vi "example_get_wavfile_amplitudes.vi"() -> ()   [LabVIEW 2017]
uses:
  <vilib>/rvi/interface/nirviOpenFPGA/nirviOpenFPGA.xnode
  <vilib>/rvi/interface/nirviCloseFPGA/nirviCloseFPGA.xnode
  <vilib>/FPGAPlugInAG/Dynamic/niLvFpga_Close_Dynamic.vi
  <vilib>/rvi/interface/nirviMethod/nirviMethod.xnode
  <vilib>/FPGAPlugInAG/Dynamic/niLvFpga_WriteFifo_Dynamic.vi
  <vilib>/rvi/errors/niLvFpgaMergeErrorWithErrorCode.vi
  FPGA Bitfiles/lab4_FPGATarget_fpgafir_PosNEB8kOJw.lvbitx
  <vilib>/FPGAPlugInAG/myRIO-1900/niLvFpga_Open_myRIO-1900.vi
  <vilib>/rvi/interface/common/dynamic/niFpgaDynamicAddResources.vi
panel:
  out "stream chart":dbl(graph)
  out "dt":dbl
  out "Wav file Amplitude graph":dbl[](graph)
  out "t0":timestamp
  out "Waveform Graph":waveform(dbl)(graph)
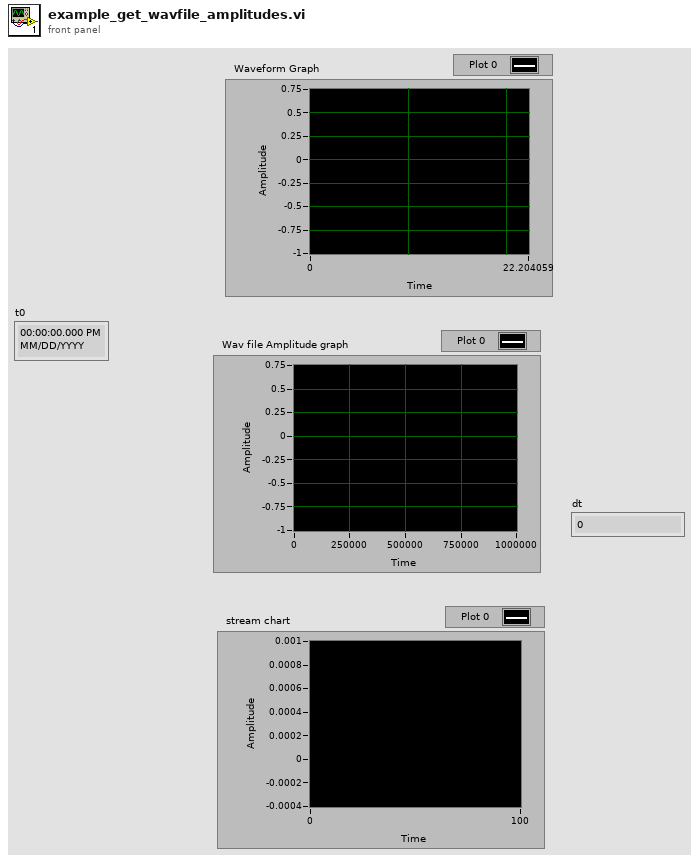
[diagram p1: front panel]
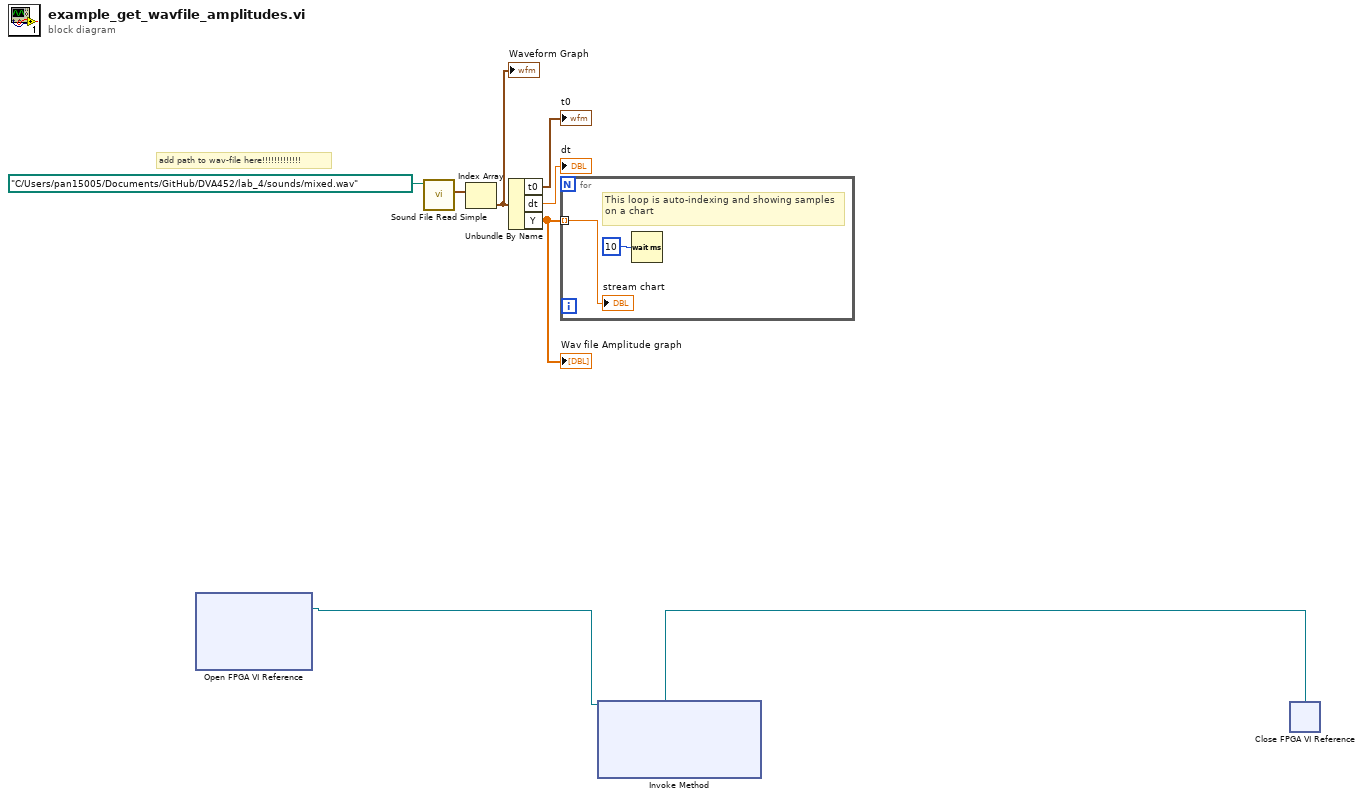
[diagram p0: block diagram]
diagram:
  # "add path to wav-file here!!!!!!!!!!!!!"
  n1 = xnode "Open FPGA VI Reference"() -> ("FPGA VI Reference Out"=w2:refnum<k20>)  [unwired: 2 in, 1 out]
  n2 = call <vilib>:"Sound File Read Simple.vi"("path"=path "C:/Users/pan15005/Documents/GitHub/DVA452/lab_4/sounds/mixed.wav") -> ("data"=w3:waveform(dbl)[])  [unwired: 7 in, 3 out]
  n3 = Index Array(array=w3) -> (element=w8:waveform(dbl))  [unwired: 1 in]
  "Waveform Graph" <- w8
  n4 = Unbundle By Name(w8) -> ("t0"=→"t0":timestamp, "dt"=→"dt":dbl, "Y"=w4:dbl[])
  "Wav file Amplitude graph" <- w4
  n5 = for {
    tunnel: w4 -> [w10] mode=indexing
    # "This loop is auto-indexing and showing samples on a chart"
    n6 = Wait (ms)(milliseconds to wait=u32 10) -> ()  [unwired: 1 out]
    "stream chart" <- w10
  }
  n7 = xnode "Invoke Method"("FPGA VI Reference In"=w2) -> ("FPGA VI Reference Out"=w1:refnum<k20>)  [unwired: 3 in, 2 out]
  n8 = xnode "Close FPGA VI Reference"("FPGA VI Reference In"=w1) -> ()  [unwired: 1 in, 1 out]
